vi "Set Compiled Code Option.vi"(8 "error in (no error)":errorcluster, 10 "Compiled code option":T1, 11 "NI_AB_API_DSDIST in":refnum<class "NI_AB_API_DSDIST.lvclass">) -> (0 "error out":errorcluster, 3 "NI_AB_API_DSDIST out":refnum<class "NI_AB_API_DSDIST.lvclass">)   [LabVIEW 2020, in "NI_AB_API_DSDIST.lvclass"]
uses:
  <vilib>/AppBuilder/AB_API/DSDIST/NI_AB_API_DSDIST.lvclass
  <vilib>/AppBuilder/AB_API/common/AB_API Compiled Code Option.ctl
  <vilib>/AppBuilder/AB_API/SDIST/NI_AB_API_SDIST.lvclass
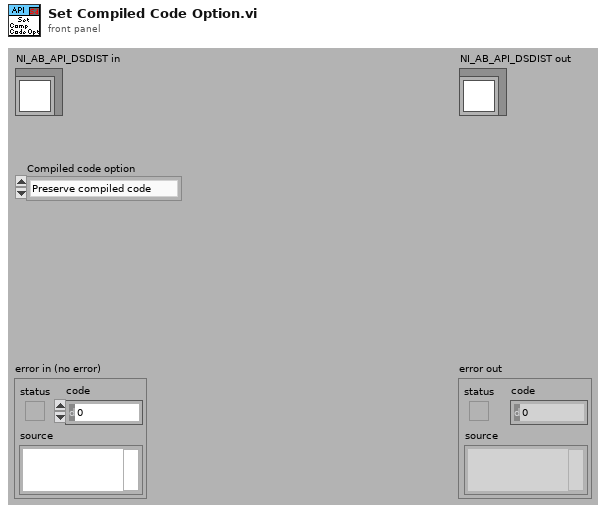
[diagram p1: front panel]
types:
  T1 = typedef "AB_API Compiled Code Option.ctl" = enum16{"Preserve compiled code", "Remove compiled code", "Preserve file settings"}
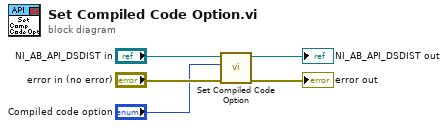
[diagram p0: block diagram]
diagram:
  n1 = call-parent "Set Compiled Code Option.vi"("error in (no error)"="error in (no error)", "Compiled code option"="Compiled code option", "NI_AB_API_SDIST in"="NI_AB_API_DSDIST in") -> ("error out"=→"error out":errorcluster, "NI_AB_API_SDIST out"=→"NI_AB_API_DSDIST out":refnum<class "NI_AB_API_DSDIST.lvclass">)  [unwired: 7 in]
